vi "Checksum.vi"(8 "Error In":errorcluster, 10 "Packet":u8[](array[numeric]), 11 "LINX Device Config":T1) -> (0 "Error Out":errorcluster, 1 "Checksum Pass?":bool, 2 "Packet":u8[](array[numeric]), 3 "LINX Device Config":T1)   [LabVIEW 2018, in "LVH-LINX.lvlib" / "Device.lvlib"]
uses:
  Device.lvlib
  Type Defs/LINX Device Config.ctl
  Type Defs/Interface.ctl
  Type Defs/TCP Config.ctl
  Type Defs/Device Family.ctl
  LVH-LINX.lvlib
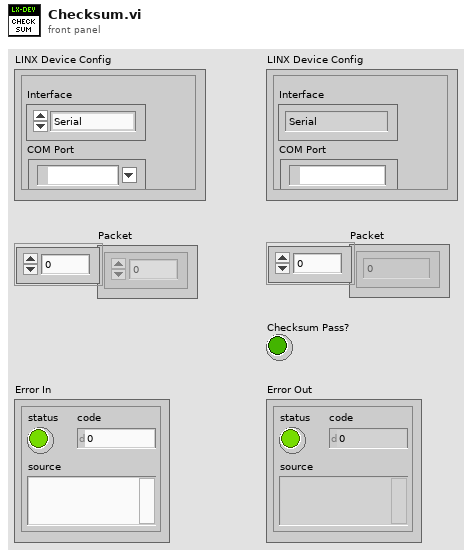
[diagram p1: front panel]
types:
  T1 = typedef "LVH-LINX.lvlib/Device.lvlib/LINX Device Config.ctl" = cluster{"Interface":T2, "COM Port":refnum<visa-resource-name>, "TCP Configuration":T3, "Device Family":T4, "Device ID":u8, "Device Name":string, "TCP Ref":refnum<k5>}
  T2 = typedef "LVH-LINX.lvlib/Interface.ctl" = enum16{"Serial", "TCP"}
  T3 = typedef "LVH-LINX.lvlib/Device.lvlib/TCP Config.ctl" = cluster{"IP Address":string, "Port":u16}
  T4 = typedef "LVH-LINX.lvlib/Device Family.ctl" = enum8{"National Instruments", "Digilent", "Arduino"}
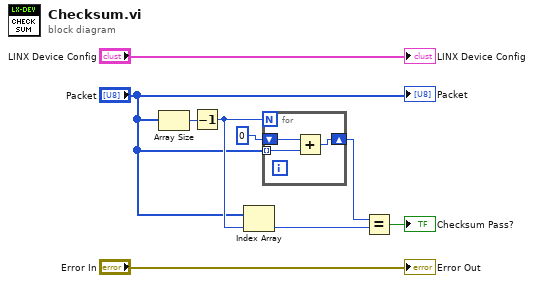
[diagram p0: block diagram]
diagram:
  n1 = Array Size(array="Packet") -> (size(s)=w9:i32)
  n2 = Decrement(x=w9) -> (x-1=w8:i32)
  n3 = Index Array(array="Packet", index=w8) -> (element=w7:u8)
  n4 = for {
    N: w8 -> [_]
    tunnel: "Packet" -> [w11] mode=indexing
    shift-right: [w10] -> w5
    shift-left: u8 0 -> [w12]
    n5 = Add(x=w12, y=w11) -> (x+y=w10:u8)
  }
  n6 = Equal?(x=w5, y=w7) -> (x = y?=→"Checksum Pass?":bool)
  "Packet" <- "Packet"
  "Error Out" <- "Error In"
  "LINX Device Config" <- "LINX Device Config"
